vi "CANAnalData.vi"(8 "error in":errorcluster, 9 "ID":u32 format="%.0x", 10 "Data":u8[](array[numeric]), 11 "Config":refnum<vi>) -> (0 "error out":errorcluster, 1 "DataLen":u8, 2 "Data out":u8[](array[numeric]), 3 "ID out":u32, 5 "TimeStamp":u32)   [LabVIEW 2017]
uses:
  PCAN_Driver/ControlCAN.llb/Return Val.ctl
  PCAN_Driver/ControlCAN.llb/VCI_CAN_OBJ.ctl
  PCAN_Driver/ControlCAN.lvlib
panel:
  out "Return Val":T1=1 items=["OK"=1, "ERROR1"=0, "ERROR2"=-1]
  in  "cnd_in":u32
  out "cnt_out":u32
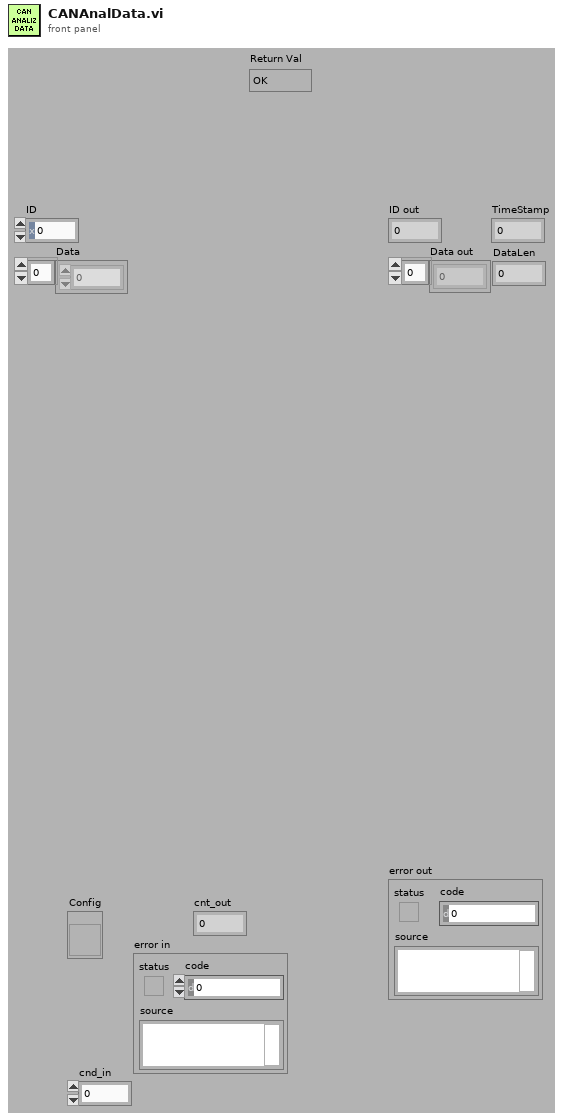
[diagram p1: front panel]
types:
  T1 = typedef "ControlCAN.lvlib/Return Val.ctl" = i32
  T2 = typedef "ControlCAN.lvlib/VCI_CAN_OBJ.ctl" = cluster{"ID":u32, "TimeStamp":u32, "TimeFlag":u8, "SendType":u8, "RemoteFlag":u8, "ExternFlag":u8, "DataLen":u8, "Data":u8[], "Reserved":u8[]}
  T3 = typedef "ControlCAN.lvlib/DevType.ctl" = u32
  T4 = typedef "ControlCAN.lvlib/CAN Channel.ctl" = u32
  T5 = typedef "ControlCAN.lvlib/VCI_INIT_CONFIG.ctl" = cluster{"AccCode":u32, "AccMask":u32, "InitFlag":T6, "Fliter":T7, "Timing0":u8, "Timing1":u8, "Mode":T8}
  T6 = typedef "ControlCAN.lvlib/InitFlag.ctl" = u32
  T7 = typedef "ControlCAN.lvlib/Fliter.ctl" = u8
  T8 = typedef "ControlCAN.lvlib/Mode.ctl" = u8
  T9 = cluster{"DevType":T3, "DevIndex":u32, "CanIndex":T4, "VCI_INIT_CONFIG":T5}
  T10 = cluster{"Type":enum16{"接收", "发送"}, "Channel":T4, "Time":timestamp, "VCI_CAN_OBJ":T2}[]
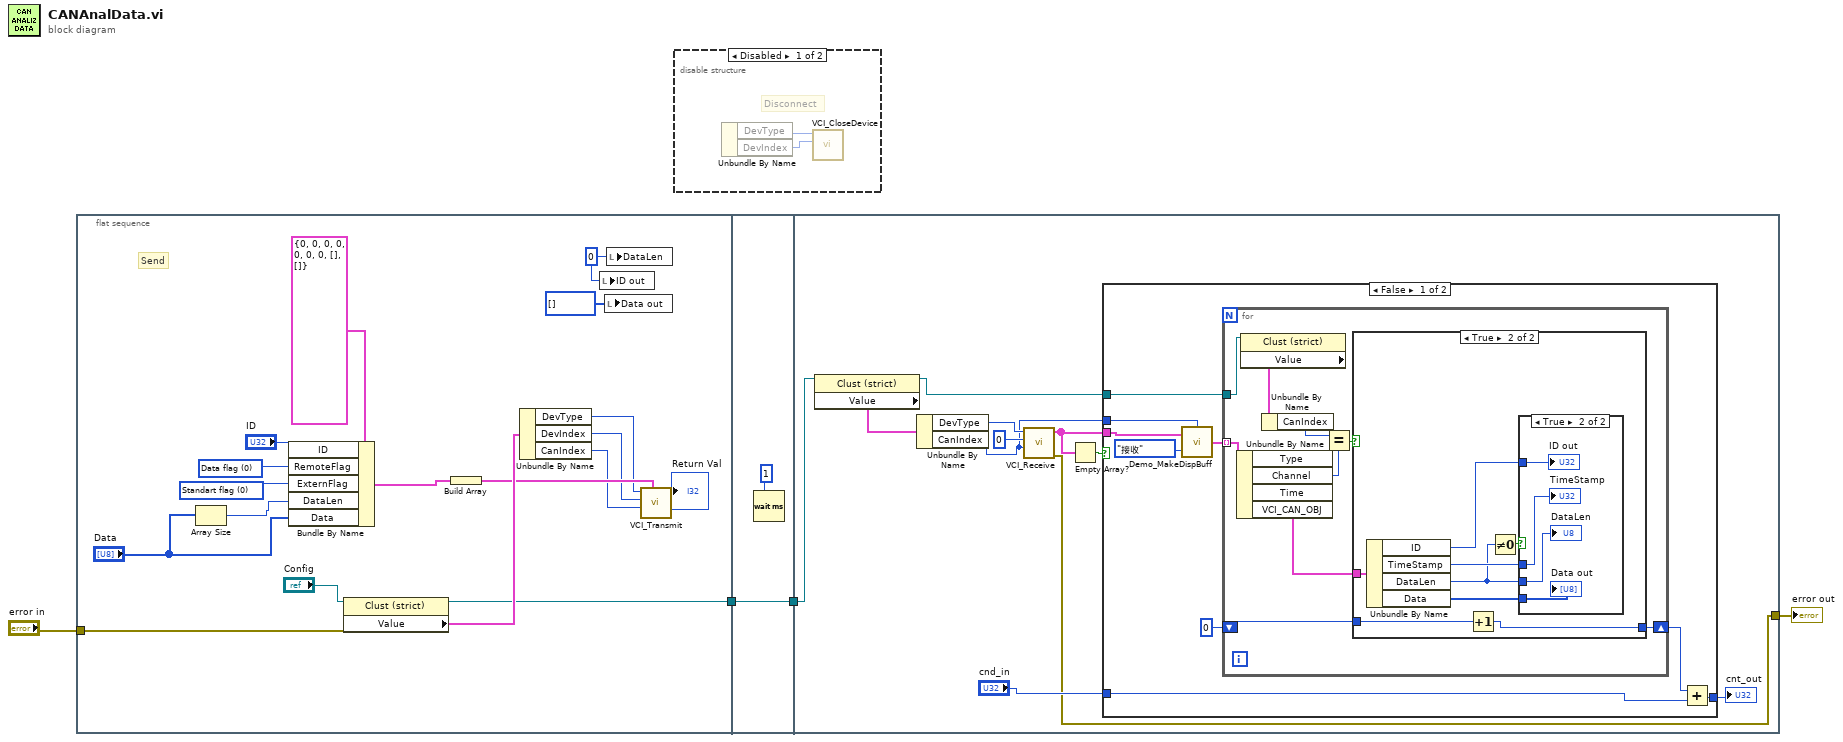
[diagram p0: block diagram]
diagram:
  n1 = flat-sequence {
    tunnel: [w9] -> w4
    tunnel: "error in" -> [w6]
    tunnel: w4 -> [w24]
    tunnel: [w24] -> w3
    tunnel: w3 -> [w26]
    tunnel: [w25] -> w1
    frame #0 {
      w8 = u8 0 ("DataLen")
      w16 = u8 0 items=["Standart flag", "Extern flag"] ("Format")
      w15 = u8 0 items=["Data flag", "Remote flag"] ("Type")
      # "Send"
      n2 = Array Size(array="Data") -> (size(s)=w11:i32)
      n3 = Bundle By Name(cluster=T2 {"ID"=0, "TimeStamp"=0, "TimeFlag"=0, "SendType"=0, "RemoteFlag"=0, "ExternFlag"=0, "DataLen"=0, "Data"=[], "Reserved"=[]} ("Send"), "ID"="ID", "RemoteFlag"=w15, "ExternFlag"=w16, "DataLen"=w11, "Data"="Data") -> (w14:T2)
      n4 = property class="Clust (strict)"(reference="Config", error in=w6) -> (reference out=w9:refnum<vi>, "Value"=w22:T9)  [unwired: 1 out]
      n5 = Build Array(w14) -> (w21:T2[])
      n6 = Unbundle By Name(w22) -> ("DevType"=w18:T3, "DevIndex"=w19:u32, "CanIndex"=w20:T4)
      n7 = local write "ID out"(w8) -> ()
      n8 = local write "Data out"(u8[] [] ("Data out")) -> ()
      n9 = local write "DataLen"(w8) -> ()
      n10 = call "VCI_Transmit.vi"("Buffer"=w21, "CANIndex"=w20, "DevIndex"=w19, "DevType"=w18) -> ("Return Val"=→"Return Val":T1)  [unwired: 1 in, 6 out]
    }
    frame #1 {
      n11 = Wait (ms)(milliseconds to wait=u32 1) -> ()  [unwired: 1 out]
    }
    frame #2 {
      n12 = property class="Clust (strict)"(reference=w26) -> (reference out=w35:refnum<vi>, "Value"=w29:T9)  [unwired: 1 in, 1 out]
      n13 = Unbundle By Name(w29) -> ("DevType"=w31:T3, "CanIndex"=w30:T4)
      n14 = call "VCI_Receive.vi"("CANIndex"=w30, "DevIndex"=u32 0, "DevType"=w31) -> ("error out"=w25:errorcluster, "Recieve"=w32:T2[])  [unwired: 3 in, 4 out]
      n15 = Empty Array?(array=w32) -> (empty?=w33:bool)
      n16 = case shown="False" w33 {
        tunnel: w32 -> [w42 _]
        tunnel: w30 -> [w43 _]
        tunnel: "cnd_in" -> [w38 w67]
        tunnel: [w37 w67] -> w28
        tunnel: w35 -> [w36 _]
        frame False {
          n17 = call "Demo_MakeDispBuff.vi"("Channel"=w43, "Type"=enum16{"接收", "发送"}."接收", "OBJs"=w42) -> ("Buffer"=w41:T10)
          n18 = for {
            tunnel: w41 -> [w53] mode=indexing
            shift-right: [w46] -> w39
            shift-left: u32 0 -> [w47]
            tunnel: w36 -> [w45]
            n19 = Unbundle By Name(w53) -> ("Channel"=w49:T4, "VCI_CAN_OBJ"=w52:T2)  [unwired: 2 out]
            n20 = property class="Clust (strict)"(reference=w45) -> ("Value"=w51:T9)  [unwired: 1 in, 2 out]
            n21 = Unbundle By Name(w51) -> ("CanIndex"=w50:T4)
            n22 = Equal?(x=w50, y=w49) -> (x = y?=w48:bool)
            n23 = case shown="True" w48 {
              tunnel: w52 -> [_ w62]
              tunnel: w47 -> [w54 w61]
              tunnel: [w54 w60] -> w46
              frame False {
              }
              frame True {
                n24 = Unbundle By Name(w62) -> ("ID"=w59:u32, "TimeStamp"=w57:u32, "DataLen"=w56:u8, "Data"=w58:u8[])
                n25 = Increment(x=w61) -> (x+1=w60:u32)
                n26 = Not Equal To 0?(x=w56) -> (x != 0?=w55:bool)
                n27 = case shown="True" w55 {
                  tunnel: w59 -> [_ w66]
                  tunnel: w58 -> [_ w65]
                  tunnel: w57 -> [_ w64]
                  tunnel: w56 -> [_ w63]
                  frame False {
                  }
                  frame True {
                    "ID out" <- w66
                    "Data out" <- w65
                    "TimeStamp" <- w64
                    "DataLen" <- w63
                  }
                }
              }
            }
          }
          n28 = Add(x=w39, y=w38) -> (x+y=w37:u32)
        }
        frame True {
        }
      }
      "cnt_out" <- w28
    }
  }
  n29 = disable-structure shown="Disabled" {
    frame Disabled {
      # "Disconnect"
      n30 = Unbundle By Name() -> ("DevType"=w69:T3, "DevIndex"=w68:u32)  [unwired: 1 in]
      n31 = call "VCI_CloseDevice.vi"("DevIndex"=w68, "DevType"=w69) -> ()  [unwired: 1 in, 9 out]
    }
    frame Enabled {
    }
  }
  "error out" <- w1
